vi "exp_DAC电压设置.vi"(1 "电压":u16, 2 "cmd_channel(8bit)":string) -> ()   [LabVIEW 2014]
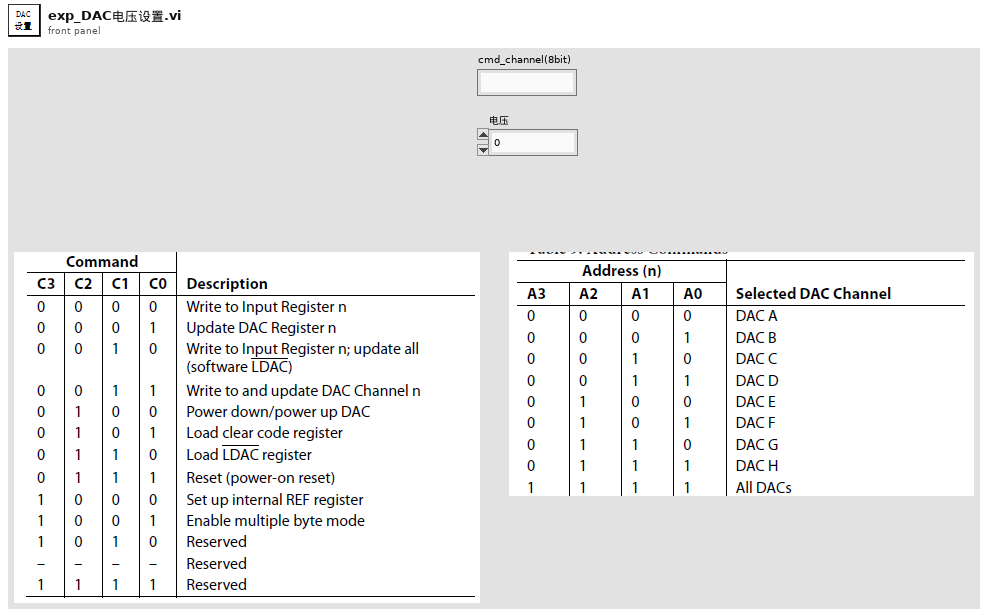
[diagram p1: front panel]
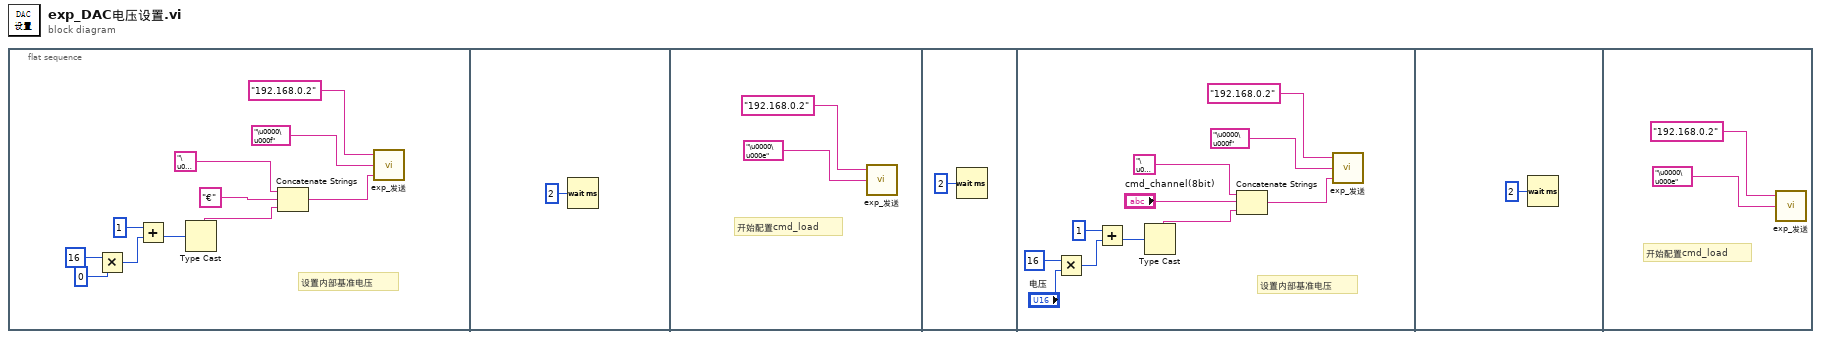
[diagram p0: block diagram]
diagram:
  n1 = flat-sequence {
    frame #0 {
      # "设置内部基准电压"
      n2 = Multiply(x=u16 16, y=u16 0) -> (x*y=w6:u16)
      n3 = Add(x=u16 1, y=w6) -> (x+y=w4:u16)
      n4 = Type Cast(x=w4) -> (*(type *) &x=w5:string)  [unwired: 1 in]
      n5 = Concatenate Strings("\u0000" ("字符串"), "€" ("字符串"), w5) -> (w9:string)
      n6 = call "exp_发送.vi"("数据（32bit）"=w9, "命令(16bit)"="\u0000\u000f", "目标IP"="192.168.0.2") -> ()  [unwired: 1 out]
    }
    frame #1 {
      n7 = Wait (ms)(milliseconds to wait=u32 2 ("等待时间（毫秒）")) -> ()  [unwired: 1 out]
    }
    frame #2 {
      # "开始配置cmd_load"
      n8 = call "exp_发送.vi"("命令(16bit)"="\u0000\u000e", "目标IP"="192.168.0.2") -> ()  [unwired: 1 in, 1 out]
    }
    frame #3 {
      n9 = Wait (ms)(milliseconds to wait=u32 2 ("等待时间（毫秒）")) -> ()  [unwired: 1 out]
    }
    frame #4 {
      # "设置内部基准电压"
      n10 = Multiply(x=u16 16, y="电压") -> (x*y=w20:u16)
      n11 = Add(x=u16 1, y=w20) -> (x+y=w18:u16)
      n12 = Type Cast(x=w18) -> (*(type *) &x=w19:string)  [unwired: 1 in]
      n13 = Concatenate Strings("\u0000" ("字符串"), "cmd_channel(8bit)", w19) -> (w24:string)
      n14 = call "exp_发送.vi"("数据（32bit）"=w24, "命令(16bit)"="\u0000\u000f", "目标IP"="192.168.0.2") -> ()  [unwired: 1 out]
    }
    frame #5 {
      n15 = Wait (ms)(milliseconds to wait=u32 2 ("等待时间（毫秒）")) -> ()  [unwired: 1 out]
    }
    frame #6 {
      # "开始配置cmd_load"
      n16 = call "exp_发送.vi"("命令(16bit)"="\u0000\u000e", "目标IP"="192.168.0.2") -> ()  [unwired: 1 in, 1 out]
    }
  }
